vi "ApplyGain - 1ch.vi"(8 "input valid":bool, 10 "gain":fxp<+/-,16,10>, 11 "data in":T2=[{"I"=0.0, "Q"=0.0, "overflow"=FALSE}]) -> (0 "output valid":bool, 3 "data out":T1[](array[typedef]))   [LabVIEW 2025]
uses:
  IQ-1element.ctl
  <instrlib>/_niInstr/DSP/v1/Shared/Public/IQ Data.ctl
  <vilib>/rvi/FXPMathLib/FxpMul/XNode/nifxpmath_Multiplier.xnode
  <vilib>/rvi/FXPMathLib/FxpConvert/XNode/nifxpmath_Convert.xnode
  <vilib>/rvi/FXPMathLib/sim/FxpSim.dll
  <vilib>/rvi/FXPMathLib/FxpConvert/simVIs/DllFxpConvertTemp_sub.vi
  <vilib>/fxp/LVFixedPointOverflowPolicyTypeDef.ctl
  <vilib>/fxp/LVFixedPointQuantizationPolicyTypeDef.ctl
  <vilib>/rvi/FXPMathLib/FxpConvert/subVIs/nifxpmath_Convert_SimConfig.ctl
  <instrlib>/_niInstr/DSP/v1/Shared/niInstr DSP v1 Shared.lvlib
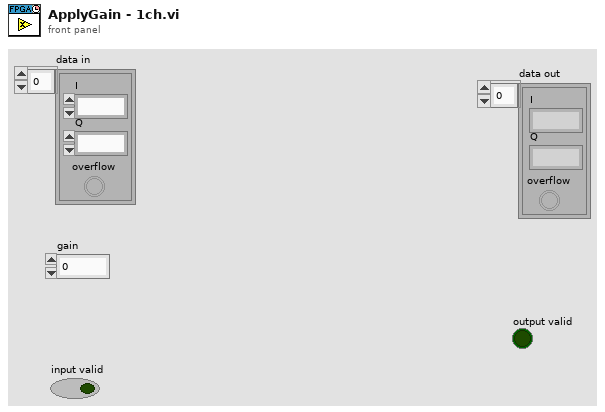
[diagram p1: front panel]
types:
  T1 = typedef "niInstr DSP v1 Shared.lvlib/IQ Data.ctl" = cluster{"I":fxp<+/-,18,1>, "Q":fxp<+/-,18,1>, "overflow":bool}
  T2 = typedef "IQ-1element.ctl" = T1[]
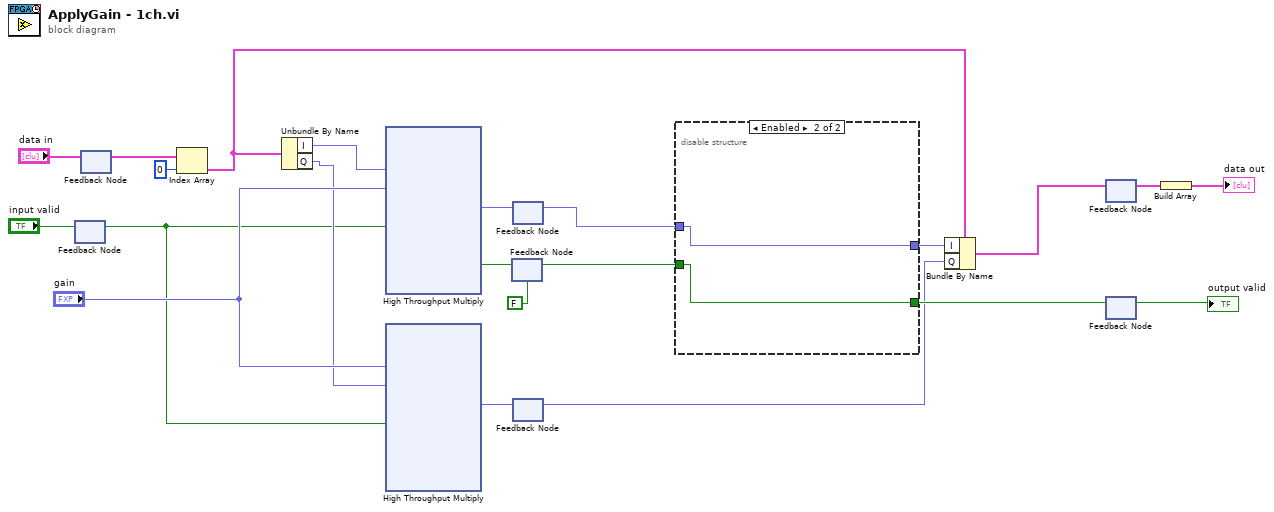
[diagram p0: block diagram]
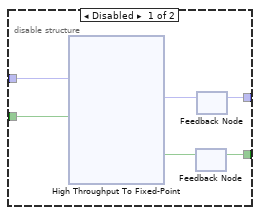
[diagram p2: hidden frame]
diagram:
  n1 = feedback #1() -> (w1:bool)  [unwired: 1 in]
  n2 = feedback-in #1("input valid") -> ()
  n3 = feedback #2() -> (w18:T2)  [unwired: 1 in]
  n4 = feedback-in #2("data in") -> ()
  n5 = Index Array(array=w18, index=0) -> (element=w12:T1)
  n6 = Unbundle By Name(w12) -> ("I"=w13:fxp<+/-,18,1>, "Q"=w3:fxp<+/-,18,1>)
  n7 = xnode ("High Throughput Multiply")("x"=w13, "y"="gain", "input valid"=w1) -> ("x*y"=w17:fxp<+/-,18,1>, "output valid"=w16:bool)  [unwired: 1 in, 1 out]
  n8 = xnode ("High Throughput Multiply")("x"="gain", "y"=w3, "input valid"=w1) -> ("x*y"=w5:fxp<+/-,18,1>)  [unwired: 1 in, 2 out]
  n9 = feedback #3(FALSE ("output valid")) -> (w14:bool)
  n10 = feedback-in #3(w16) -> ()
  n11 = feedback #4() -> (w6:fxp<+/-,18,1>)  [unwired: 1 in]
  n12 = feedback-in #4(w17) -> ()
  n13 = feedback #5() -> (w2:fxp<+/-,18,1>)  [unwired: 1 in]
  n14 = feedback-in #5(w5) -> ()
  n15 = disable-structure shown="Enabled" {
    disable-tunnel: w14 -> [w28 w53]
    disable-tunnel: [w25 w54] -> w11
    disable-tunnel: [w24 w53] -> w8
    disable-tunnel: w6 -> [w23 w54]
    frame Disabled {
      n16 = xnode "High Throughput To Fixed-Point"("x"=w23, "input valid"=w28) -> ("y"=w27:fxp<+/-,18,1>, "output valid"=w26:bool)  [unwired: 1 in, 1 out]
      n17 = feedback #6() -> (w24:bool)  [unwired: 1 in]
      n18 = feedback-in #6(w26) -> ()
      n19 = feedback #7() -> (w25:fxp<+/-,18,1>)  [unwired: 1 in]
      n20 = feedback-in #7(w27) -> ()
    }
    frame Enabled {
    }
  }
  n21 = Bundle By Name(cluster=w12, "I"=w11, "Q"=w2) -> (w10:T1)
  n22 = feedback #8() -> (w21:T1)  [unwired: 1 in]
  n23 = feedback-in #8(w10) -> ()
  n24 = feedback #9() -> (→"output valid":bool)  [unwired: 1 in]
  n25 = feedback-in #9(w8) -> ()
  n26 = Build Array(w21) -> (→"data out":T1[])
